vi "Set All Filters.vi"(8 "error in (no error)":errorcluster, 10 "Filter Wheel Position":i32[](array[numeric]), 11 "Filter Wheel in":refnum<class "Filter Wheel.lvclass">) -> (0 "error out":errorcluster, 3 "Filter Wheel out":refnum<class "Filter Wheel.lvclass">)   [LabVIEW 2024, in "Filter Wheel.lvclass"]
uses:
  Filter Wheel Object/Filter Wheel.lvclass
  Filter Wheel Object/Filter Wheel.lvclass/Filter Wheel.ctl
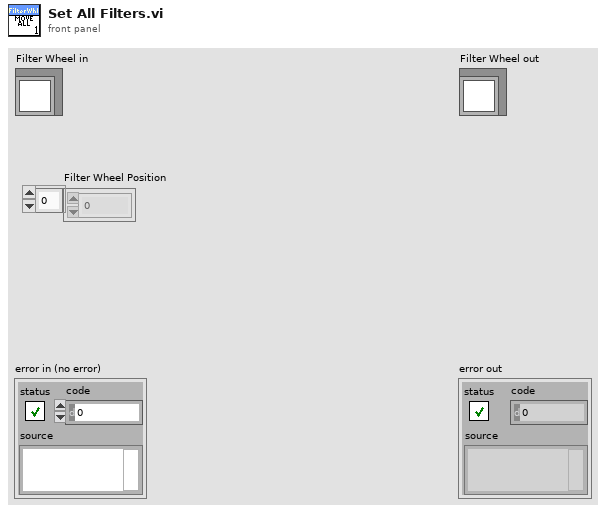
[diagram p1: front panel]
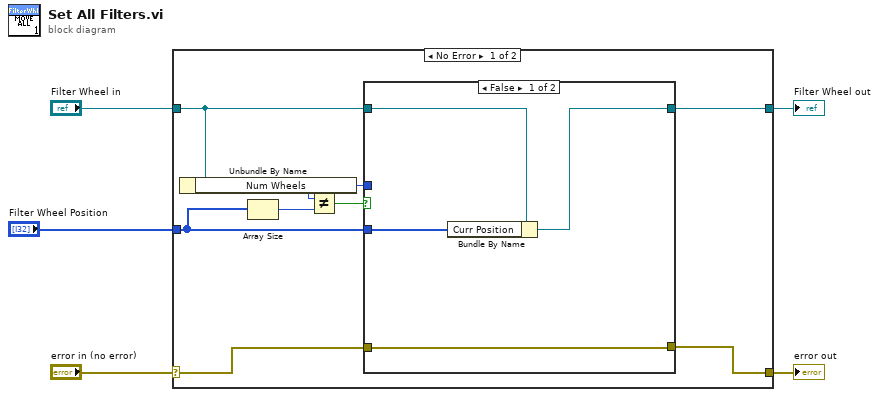
[diagram p0: block diagram]
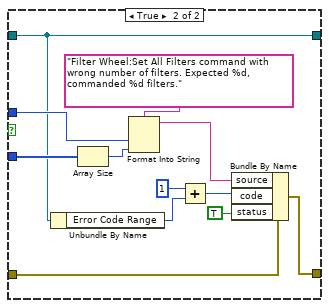
[diagram p2: hidden frame]
diagram:
  n1 = case shown="No Error" "error in (no error)" {
    selector: "error in (no error)" -> [w11 w31]
    tunnel: [w6 w31] -> w4
    tunnel: [w8 w30] -> w1
    tunnel: "Filter Wheel in" -> [w10 w30]
    tunnel: "Filter Wheel Position" -> [w9 _]
    frame No Error {
      n2 = Unbundle By Name(w10) -> ("Num Wheels"=w7:i32)
      n3 = Array Size(array=w9) -> (size(s)=w13:i32)
      n4 = Not Equal?(x=w7, y=w13) -> (x != y?=w12:bool)
      n5 = case shown="False" w12 {
        tunnel: w11 -> [w14 w29]
        tunnel: w10 -> [w17 w23]
        tunnel: w9 -> [w16 w27]
        tunnel: [w15 w23] -> w8
        tunnel: w7 -> [_ w25]
        tunnel: [w14 w18] -> w6
        frame False {
          n6 = Bundle By Name(cluster=w17, "Curr Position"=w16) -> (w15:refnum<class "Filter Wheel.lvclass">)
        }
        frame True {
          n7 = Unbundle By Name(w23) -> ("Error Code Range"=w22:i32)
          n8 = Array Size(array=w27) -> (size(s)=w26:i32)
          n9 = Format Into String(format string="Filter Wheel:Set All Filters command with wrong number of filters. Expected %d, commanded %d filters.", w25, w26) -> (resulting string=w24:string)  [unwired: 2 in, 1 out]
          n10 = Add(x=1, y=w22) -> (x+y=w20:i32)
          n11 = Bundle By Name(cluster=w29, "source"=w24, "code"=w20, "status"=TRUE) -> (w18:errorcluster)
        }
      }
    }
    frame Error {
    }
  }
  "error out" <- w4
  "Filter Wheel out" <- w1
